vi "String_2_Number.vi"(1 "Value":string) -> (0 "Numeric":dbl)   [LabVIEW 2011]
doc: "Replaces any commas in value string with decimal points, prior to converting to DBL. (Don't know why...! TCRL)"
panel:
  # "Replaces any commas in value string with decimal points,\nprior to converting to DBL"
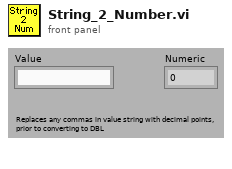
[diagram p1: front panel]
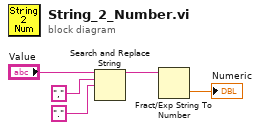
[diagram p0: block diagram]
diagram:
  n1 = Search and Replace String(input string="Value", search string=",", replace string="." ("replace string (\"\")")) -> (result string=w5:string)  [unwired: 5 in, 3 out]
  n2 = Fract/Exp String To Number(string=w5) -> (number=→"Numeric":dbl)  [unwired: 4 out]
